vi "LVIS_Initialize.vi"(8 "Error In":errorcluster, 11 "Validate?":bool) -> (0 "Error Out":errorcluster, 3 "Success?":bool)   [LabVIEW 2015]
doc: "Initializes variables, reads the configuration file and verifies the content, checks the DC connection, launches the Status Process and, if enabled, launches the Event Log."
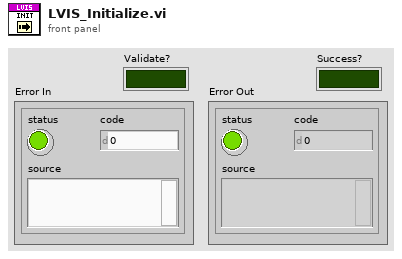
[diagram p1: front panel]
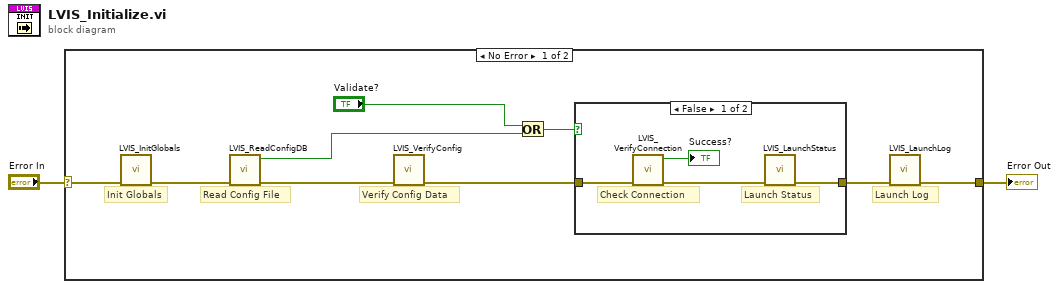
[diagram p0: block diagram]
diagram:
  n1 = case shown="No Error" "Error In" {
    selector: "Error In" -> [w11 w17]
    tunnel: [w6 w17] -> w1
    frame No Error {
      # "Read Config File"
      # "Launch Log"
      # "Verify Config Data"
      # "Init Globals"
      n2 = call "LVIS_InitGlobals.vi"("Error In"=w11) -> ("Error Out"=w10:errorcluster)  [unwired: 10 in]
      n3 = call "LVIS_ReadConfigDB.vi"("Error In"=w10) -> ("Error Out"=w9:errorcluster, "Disable"=w3:bool)  [unwired: 9 in]
      n4 = call "LVIS_VerifyConfig.vi"("Error In"=w9) -> ("Error Out"=w8:errorcluster)  [unwired: 10 in]
      n5 = Or(x="Validate?", y=w3) -> (x .or. y?=w5:bool)
      n6 = case shown="False" w5 {
        tunnel: [w15 w16] -> w7
        tunnel: w8 -> [w12 w16]
        frame False {
          # "Launch Status"
          # "Check Connection"
          n7 = call "LVIS_VerifyConnection.vi"("Error In"=w12) -> ("Error Out"=w13:errorcluster, "Success?"=→"Success?":bool)  [unwired: 9 in]
          n8 = call "LVIS_LaunchStatus.vi"("Error In"=w13) -> ("Error Out"=w15:errorcluster)  [unwired: 10 in]
        }
        frame True {
          # "Data Commander has been disabled"
        }
      }
      n9 = call "LVIS_LaunchLog.vi"("Error In"=w7) -> ("Error Out"=w6:errorcluster)  [unwired: 10 in]
    }
    frame Error {
    }
  }
  "Error Out" <- w1
